vi "DRAM FIFO test with data.vi"() -> ()   [LabVIEW 2019]
uses:
  <instrlib>/FlexRIO/DRAM FIFO/v2/FPGA/DRAM FIFO/DRAM FIFO Status.ctl
  <instrlib>/FlexRIO/DRAM FIFO/v2/FPGA/DRAM FIFO/FIFO Depth.ctl
  <vilib>/Platform/TimedLoop/XDataNode/timing_clust.ctl
  <vilib>/Platform/TimedLoop/XDataNode/nitl_modes.ctl
  <vilib>/Platform/TimedLoop/XDataNode/wakeup.ctl
  <instrlib>/FlexRIO/DRAM FIFO/v2/FPGA/DRAM FIFO/dynamic arbitration select.ctl
  <instrlib>/FlexRIO/DRAM FIFO/v2/FPGA/DRAM FIFO/Private/DRAM FIFO U512/Create 512x1 DRAM FIFO.vi
  <vilib>/rvi/Emulation/niFpgaSctlEmulationGetInTimedLoop.vi
  <vilib>/rvi/Emulation/niFpgaEmulationReportErrorSimple.vi
  <vilib>/rvi/Emulation/niFpgaGetClockAttributes.vi
  <vilib>/rvi/Emulation/niFpgaCriticalErrorInLSC.vi
  <vilib>/rvi/Emulation/niFpgaProcessEmulError.vi
  <instrlib>/_niInstr/Basic Elements/v1/FPGA/Private/Count Up U32.vi
  <instrlib>/_niInstr/Basic Elements/v1/FPGA/Private/Count Up U16.vi
  <instrlib>/_niInstr/Data Formatting/v1/FPGA/Private/Convert/FXP(+-,12,1) array to Boolean Array.vi
  <instrlib>/_niInstr/Basic Elements/v1/FPGA/Private/Count Down U32.vi
  <instrlib>/FlexRIO/DRAM FIFO/v2/FPGA/DRAM FIFO/Pack Boolean Array.vi
  <vilib>/rvi/interface/RandomDataEmulation/nirviRandomDataMultiElementFPGAFIFO.vi
  <instcachedir>/0/nirviRandomDataMultiElementFPGAFIFO_1ED88BA00AC641F388A9B1FAA20E354D.lvgen/nirviRandomDataMultiElementFPGAFIFO_1ED88BA00AC641F388A9B1FAA20E354D_003.vi
  <vilib>/rvi/interface/RandomDataEmulation/niFpgaRandomDataHandleErrors.vi
  <vilib>/platform/TimedLoop/XDataNode/XDataNode.xnode
  <vilib>/rvi/FXPMathLib/FxpInterpret/XNode/nifxpmath_Interpret.xnode
  <vilib>/rvi/DataTransferAndStorage/Container/XNode/niFpgaContainer.xnode
  <vilib>/rvi/interface/RandomDataEmulation/nirviRandomDataFpgaMultiElementTemplate.vi
  <instrlib>/FlexRIO/DRAM FIFO/v2/FPGA/DRAM FIFO/DRAM FIFO v2 FPGA.lvclass
  <vilib>/Platform/TimedLoop/XDataNode/XDNodeRunTimeDep.lvlib
  <instrlib>/_niInstr/Data Formatting/v1/FPGA/niInstr Data Formatting v1 FPGA.lvlib
  <instrlib>/_niInstr/Basic Elements/v1/FPGA/niInstr Basic Elements v1 FPGA.lvlib
  SubVIs/Utility/FPGA Utility.lvlib
  <instrlib>/FlexRIO/DRAM FIFO/v2/FPGA/DRAM FIFO/Private/DRAM FIFO U512/DRAM FIFO U512 v2 FPGA.lvclass
panel:
  out "DRAM writes ctr":u32
  out "dram full latch":bool
  out "DRAM highwater 2":u32
  out "acq active":bool
  in  "start":bool
  in  "signal length":u32
  out "DRAM overflow":bool
  out "DRAM highwater":u32
  out "reset in progress?":bool
  in  "reset DRAM":bool
  out "status":T1
  in  "reset":bool
  in  "dram.flush":bool
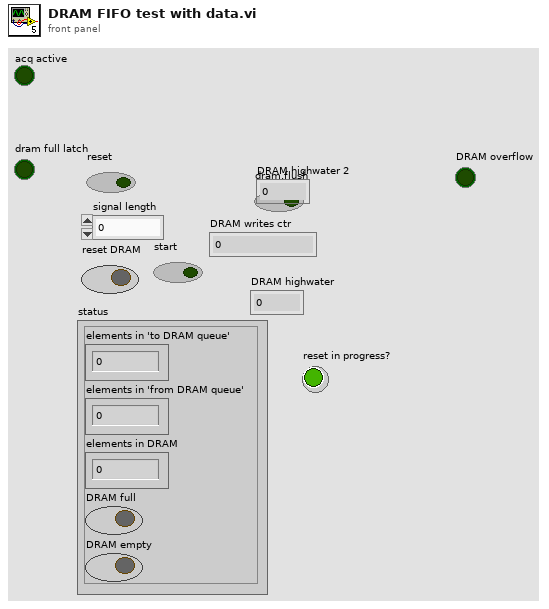
[diagram p1: front panel]
types:
  T1 = typedef "DRAM FIFO v2 FPGA.lvclass/DRAM FIFO Status.ctl" = cluster{"elements in 'to DRAM queue'":u32, "elements in 'from DRAM queue'":u32, "elements in DRAM":u32, "DRAM full":bool, "DRAM empty":bool}
  T2 = typedef "DRAM FIFO v2 FPGA.lvclass/FIFO Depth.ctl" = u8
  T3 = typedef "XDNodeRunTimeDep.lvlib/timing_clust.ctl" = cluster{"Expected End [f-1]":u64, "Actual End [f-1]":u64, "Finished Late? [f-1]":bool, "Expected End [i-1]":u64, "Actual End [i-1]":u64, "Finished Late? [i-1]":bool, "Expected Start [i]":u64, "Actual Start [i]":u64, "Expected Start [f]":u64, "Actual Start [f]":u64, "Source Name":string, "Structure Name":string, "Period":i64, "Deadline":i64, "Offset":i64, "Start":i64, "Priority":i32, "Timeout":i32, "Mode":T4, "Wakeup Reason":T5, "Error":errorcluster, "Source Type":string, "Secondary Source Type":string, "Global End Time":u64, "Global Start Time":u64, "Frame Duration":u64, "Iteration Duration":u64, "Assigned CPU":i32, "I/O Scan Engine Mode":u32}
  T4 = typedef "XDNodeRunTimeDep.lvlib/nitl_modes.ctl" = enum32{"No Change", "Process missed periods, maintain original phase", "Discard missed periods, maintain original phase", "Process missed periods, ignore original phase", "Discard missed periods, ignore original phase"}
  T5 = typedef "XDNodeRunTimeDep.lvlib/wakeup.ctl" = enum32{"Normal", "Aborted", "Asynchronous wakeup", "Timing source error", "Timed loop error", "Timeout"}
  T6 = typedef "DRAM FIFO v2 FPGA.lvclass/dynamic arbitration select.ctl" = enum16{"none", "dynamic (priority writes)", "dynamic (priority reads)"}
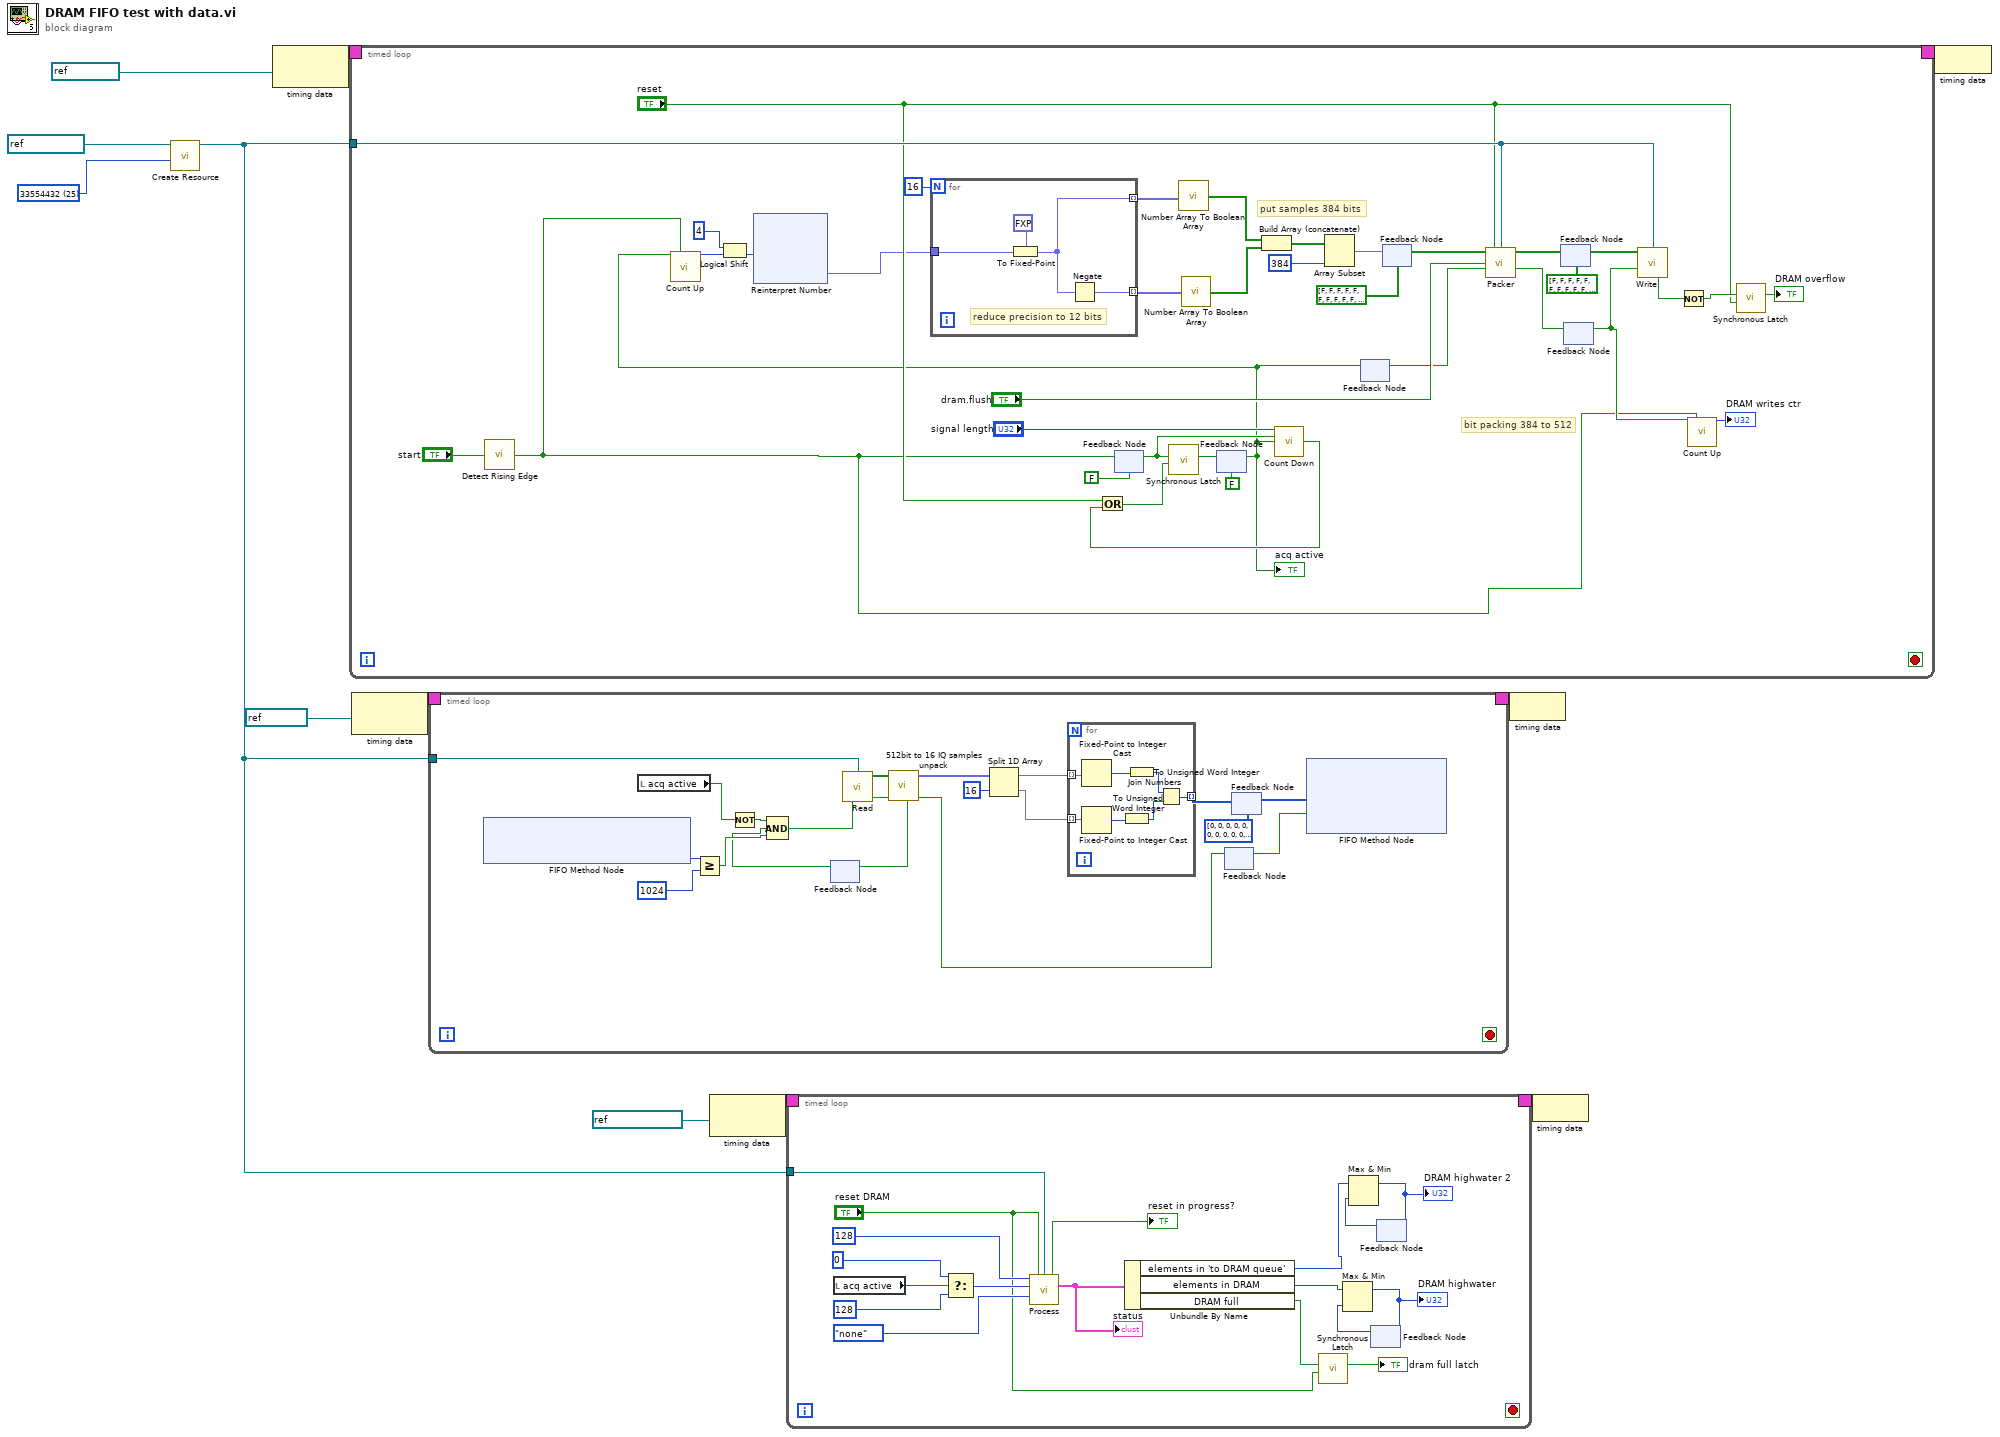
[diagram p0: block diagram]
diagram:
  w9 = T2 25 items=["4"=2, "8"=3, "16"=4, "32"=5, "64"=6, "128"=7, "256"=8, "512"=9, "1024"=10, "2048"=11, "4096"=12, "8192"=13, "16384"=14, "32768"=15, "65536"=16, "131072"=17, "262144"=18, "524288"=19, "1048576"=20, "2097152"=21, "4194304"=22, "8388608"=23, "16777216"=24, "33554432"=25, "67108864"=26, "134217728"=27, "268435456"=28, "536870912"=29, "1073741824"=30, "2147483648"=31, "4294967296"=32] ("actual # of DRAM elements")
  n1 = call-poly <instrlib>:"Create Resource.vi"("actual # of DRAM elements"=w9, "memory refnum"=refnum<k21> "RX memo") -> ("DRAM FIFO ref out"=w1:refnum<class "DRAM FIFO v2 FPGA.lvclass">)  [unwired: 9 in]
  n2 = node-c288(refnum<k21> "192MHz" ("Source Name")) -> (w7:T3)
  n3 = timed-loop {
    timing: w7 -> [_]
    timing-out: [_] -> w6
    tunnel: w1 -> [w32]
    stop <- _ stop-if-true
    # "bit packing 384 to 512"
    # "put samples 384 bits"
    n4 = call <instrlib>:"Detect Rising Edge.vi"("signal"="start") -> ("edge detected"=w14:bool)  [unwired: 14 in]
    n5 = feedback #1(FALSE ("edge detected")) -> (w36:bool)
    n6 = feedback-in #1(w14) -> ()
    n7 = feedback #2(FALSE ("out")) -> (w21:bool)
    "acq active" <- w21
    n8 = call-poly <instrlib>:"Count Up.vi"("increment"=w21, "reset"=w14) -> ("count out"=w19:u16)  [unwired: 13 in]
    n9 = Logical Shift(y=i16 4, x=w19) -> (x << y=w17:u16)
    n10 = xnode "Reinterpret Number"("x"=w17) -> ("y"=w18:fxp<+/-,16,1>)
    n11 = for {
      N: 16 -> [_]
      tunnel: [w50] -> w46 mode=indexing
      tunnel: [w52] -> w42 mode=indexing
      tunnel: w18 -> [w51]
      # "reduce precision to 12 bits"
      n12 = To Fixed-Point(fixed-point type=fxp<+/-,12,1> 0.0, number=w51) -> (fixed-point=w50:fxp<+/-,12,1>)
      n13 = Negate(x=w50) -> (-x=w52:fxp<+/-,12,1>)
    }
    n14 = call-poly <instrlib>:"Number Array To Boolean Array.vi"("data in"=w46) -> ("data out"=w45:bool[])  [unwired: 14 in]
    n15 = call-poly <instrlib>:"Number Array To Boolean Array.vi"("data in"=w42) -> ("data out"=w41:bool[])  [unwired: 14 in]
    n16 = Build Array (concatenate)(w45, w41) -> (w43:bool[])
    n17 = call-poly <instrlib>:"Count Down.vi"("count in"="signal length", "load"=w36, "decrement"=w21) -> ("terminal count"=w31:bool)  [unwired: 11 in, 1 out]
    n18 = Or(x="reset", y=w31) -> (x .or. y?=w30:bool)
    n19 = call <instrlib>:"Synchronous Latch.vi"("clear"=w30, "set"=w36) -> ("out"=w29:bool)  [unwired: 9 in]
    n20 = feedback-in #2(w29) -> ()
    n21 = Array Subset(array=w43, length=384) -> (w28:bool[])  [unwired: 1 in]
    n22 = feedback #3() -> (w25:bool)  [unwired: 1 in]
    n23 = feedback-in #3(w21) -> ()
    n24 = feedback #4(bool[] [FALSE, FALSE, FALSE, FALSE, FALSE, FALSE, FALSE, FALSE, FALSE, FALSE, FALSE, FALSE, FALSE, FALSE, FALSE, FALSE, FALSE, FALSE, FALSE, FALSE, FALSE, FALSE, FALSE, FALSE, FALSE, FALSE, FALSE, FALSE, FALSE, FALSE, FALSE, FALSE, FALSE, FALSE, FALSE, FALSE, FALSE, FALSE, FALSE, FALSE, FALSE, FALSE, FALSE, FALSE, FALSE, FALSE, FALSE, FALSE, FALSE, FALSE, FALSE, FALSE, FALSE, FALSE, FALSE, FALSE, FALSE, FALSE, FALSE, FALSE, FALSE, FALSE, FALSE, FALSE, FALSE, FALSE, FALSE, FALSE, FALSE, FALSE, FALSE, FALSE, FALSE, FALSE, FALSE, FALSE, FALSE, FALSE, FALSE, FALSE, FALSE, FALSE, FALSE, FALSE, FALSE, FALSE, FALSE, FALSE, FALSE, FALSE, FALSE, FALSE, FALSE, FALSE, FALSE, FALSE, FALSE, FALSE, FALSE, FALSE, FALSE, FALSE, FALSE, FALSE, FALSE, FALSE, FALSE, FALSE, FALSE, FALSE, FALSE, FALSE, FALSE, FALSE, FALSE, FALSE, FALSE, FALSE, FALSE, FALSE, FALSE, FALSE, FALSE, FALSE, FALSE, FALSE, FALSE, FALSE, FALSE, FALSE, FALSE, FALSE, FALSE, FALSE, FALSE, FALSE, FALSE, FALSE, FALSE, FALSE, FALSE, FALSE, FALSE, FALSE, FALSE, FALSE, FALSE, FALSE, FALSE, FALSE, FALSE, FALSE, FALSE, FALSE, FALSE, FALSE, FALSE, FALSE, FALSE, FALSE, FALSE, FALSE, FALSE, FALSE, FALSE, FALSE, FALSE, FALSE, FALSE, FALSE, FALSE, FALSE, FALSE, FALSE, FALSE, FALSE, FALSE, FALSE, FALSE, FALSE, FALSE, FALSE, FALSE, FALSE, FALSE, FALSE, FALSE, FALSE, FALSE, FALSE, FALSE, FALSE, FALSE, FALSE, FALSE, FALSE, FALSE, FALSE, FALSE, FALSE, FALSE, FALSE, FALSE, FALSE, FALSE, FALSE, FALSE, FALSE, FALSE, FALSE, FALSE, FALSE, FALSE, FALSE, FALSE, FALSE, FALSE, FALSE, FALSE, FALSE, FALSE, FALSE, FALSE, FALSE, FALSE, FALSE, FALSE, FALSE, FALSE, FALSE, FALSE, FALSE, FALSE, FALSE, FALSE, FALSE, FALSE, FALSE, FALSE, FALSE, FALSE, FALSE, FALSE, FALSE, FALSE, FALSE, FALSE, FALSE, FALSE, FALSE, FALSE, FALSE, FALSE, FALSE, FALSE, FALSE, FALSE, FALSE, FALSE, FALSE, FALSE, FALSE, FALSE, FALSE, FALSE, FALSE, FALSE, FALSE, FALSE, FALSE, FALSE, FALSE, FALSE, FALSE, FALSE, FALSE, FALSE, FALSE, FALSE, FALSE, FALSE, FALSE, FALSE, FALSE, FALSE, FALSE, FALSE, FALSE, FALSE, FALSE, FALSE, FALSE, FALSE, FALSE, FALSE, FALSE, FALSE, FALSE, FALSE, FALSE, FALSE, FALSE, FALSE, FALSE, FALSE, FALSE, FALSE, FALSE, FALSE, FALSE, FALSE, FALSE, FALSE, FALSE, FALSE, FALSE, FALSE, FALSE, FALSE, FALSE, FALSE, FALSE, FALSE, FALSE, FALSE, FALSE, FALSE, FALSE, FALSE, FALSE, FALSE, FALSE, FALSE, FALSE, FALSE, FALSE, FALSE, FALSE, FALSE, FALSE, FALSE, FALSE, FALSE, FALSE, FALSE, FALSE, FALSE, FALSE, FALSE, FALSE, FALSE, FALSE, FALSE, FALSE, FALSE, FALSE, FALSE, FALSE, FALSE, FALSE, FALSE, FALSE, FALSE, FALSE, FALSE, FALSE, FALSE, FALSE, FALSE, FALSE, FALSE, FALSE, FALSE, FALSE, FALSE, FALSE, FALSE, FALSE, FALSE, FALSE, FALSE, FALSE, FALSE, FALSE]) -> (w27:bool[])
    n25 = feedback-in #4(w28) -> ()
    n26 = call-poly <instrlib>:"Packer.vi"("data in"=w27, "reset"="reset", "DRAM FIFO in"=w32, "flush data"="dram.flush", "input valid"=w25) -> ("data out"=w47:bool[], "output valid"=w48:bool)  [unwired: 8 in, 1 out]
    n27 = feedback #5(bool[] [FALSE, FALSE, FALSE, FALSE, FALSE, FALSE, FALSE, FALSE, FALSE, FALSE, FALSE, FALSE, FALSE, FALSE, FALSE, FALSE, FALSE, FALSE, FALSE, FALSE, FALSE, FALSE, FALSE, FALSE, FALSE, FALSE, FALSE, FALSE, FALSE, FALSE, FALSE, FALSE, FALSE, FALSE, FALSE, FALSE, FALSE, FALSE, FALSE, FALSE, FALSE, FALSE, FALSE, FALSE, FALSE, FALSE, FALSE, FALSE, FALSE, FALSE, FALSE, FALSE, FALSE, FALSE, FALSE, FALSE, FALSE, FALSE, FALSE, FALSE, FALSE, FALSE, FALSE, FALSE, FALSE, FALSE, FALSE, FALSE, FALSE, FALSE, FALSE, FALSE, FALSE, FALSE, FALSE, FALSE, FALSE, FALSE, FALSE, FALSE, FALSE, FALSE, FALSE, FALSE, FALSE, FALSE, FALSE, FALSE, FALSE, FALSE, FALSE, FALSE, FALSE, FALSE, FALSE, FALSE, FALSE, FALSE, FALSE, FALSE, FALSE, FALSE, FALSE, FALSE, FALSE, FALSE, FALSE, FALSE, FALSE, FALSE, FALSE, FALSE, FALSE, FALSE, FALSE, FALSE, FALSE, FALSE, FALSE, FALSE, FALSE, FALSE, FALSE, FALSE, FALSE, FALSE, FALSE, FALSE, FALSE, FALSE, FALSE, FALSE, FALSE, FALSE, FALSE, FALSE, FALSE, FALSE, FALSE, FALSE, FALSE, FALSE, FALSE, FALSE, FALSE, FALSE, FALSE, FALSE, FALSE, FALSE, FALSE, FALSE, FALSE, FALSE, FALSE, FALSE, FALSE, FALSE, FALSE, FALSE, FALSE, FALSE, FALSE, FALSE, FALSE, FALSE, FALSE, FALSE, FALSE, FALSE, FALSE, FALSE, FALSE, FALSE, FALSE, FALSE, FALSE, FALSE, FALSE, FALSE, FALSE, FALSE, FALSE, FALSE, FALSE, FALSE, FALSE, FALSE, FALSE, FALSE, FALSE, FALSE, FALSE, FALSE, FALSE, FALSE, FALSE, FALSE, FALSE, FALSE, FALSE, FALSE, FALSE, FALSE, FALSE, FALSE, FALSE, FALSE, FALSE, FALSE, FALSE, FALSE, FALSE, FALSE, FALSE, FALSE, FALSE, FALSE, FALSE, FALSE, FALSE, FALSE, FALSE, FALSE, FALSE, FALSE, FALSE, FALSE, FALSE, FALSE, FALSE, FALSE, FALSE, FALSE, FALSE, FALSE, FALSE, FALSE, FALSE, FALSE, FALSE, FALSE, FALSE, FALSE, FALSE, FALSE, FALSE, FALSE, FALSE, FALSE, FALSE, FALSE, FALSE, FALSE, FALSE, FALSE, FALSE, FALSE, FALSE, FALSE, FALSE, FALSE, FALSE, FALSE, FALSE, FALSE, FALSE, FALSE, FALSE, FALSE, FALSE, FALSE, FALSE, FALSE, FALSE, FALSE, FALSE, FALSE, FALSE, FALSE, FALSE, FALSE, FALSE, FALSE, FALSE, FALSE, FALSE, FALSE, FALSE, FALSE, FALSE, FALSE, FALSE, FALSE, FALSE, FALSE, FALSE, FALSE, FALSE, FALSE, FALSE, FALSE, FALSE, FALSE, FALSE, FALSE, FALSE, FALSE, FALSE, FALSE, FALSE, FALSE, FALSE, FALSE, FALSE, FALSE, FALSE, FALSE, FALSE, FALSE, FALSE, FALSE, FALSE, FALSE, FALSE, FALSE, FALSE, FALSE, FALSE, FALSE, FALSE, FALSE, FALSE, FALSE, FALSE, FALSE, FALSE, FALSE, FALSE, FALSE, FALSE, FALSE, FALSE, FALSE, FALSE, FALSE, FALSE, FALSE, FALSE, FALSE, FALSE, FALSE, FALSE, FALSE, FALSE, FALSE, FALSE, FALSE, FALSE, FALSE, FALSE, FALSE, FALSE, FALSE, FALSE, FALSE, FALSE, FALSE, FALSE, FALSE, FALSE, FALSE, FALSE, FALSE, FALSE, FALSE, FALSE, FALSE, FALSE, FALSE, FALSE, FALSE, FALSE, FALSE, FALSE, FALSE, FALSE, FALSE, FALSE, FALSE, FALSE, FALSE, FALSE, FALSE, FALSE, FALSE, FALSE, FALSE, FALSE, FALSE, FALSE, FALSE, FALSE, FALSE, FALSE, FALSE, FALSE, FALSE, FALSE, FALSE, FALSE, FALSE, FALSE, FALSE, FALSE, FALSE, FALSE, FALSE, FALSE, FALSE, FALSE, FALSE, FALSE, FALSE, FALSE, FALSE, FALSE, FALSE, FALSE, FALSE, FALSE, FALSE, FALSE, FALSE, FALSE, FALSE, FALSE, FALSE, FALSE, FALSE, FALSE, FALSE, FALSE, FALSE, FALSE, FALSE, FALSE, FALSE, FALSE, FALSE, FALSE, FALSE, FALSE, FALSE, FALSE, FALSE, FALSE, FALSE, FALSE, FALSE, FALSE, FALSE, FALSE, FALSE, FALSE, FALSE, FALSE, FALSE, FALSE, FALSE, FALSE, FALSE, FALSE, FALSE, FALSE, FALSE, FALSE, FALSE, FALSE, FALSE, FALSE, FALSE, FALSE, FALSE, FALSE, FALSE, FALSE, FALSE, FALSE, FALSE, FALSE, FALSE, FALSE, FALSE, FALSE, FALSE, FALSE, FALSE, FALSE, FALSE, FALSE, FALSE, FALSE, FALSE, FALSE, FALSE, FALSE, FALSE, FALSE, FALSE, FALSE, FALSE]) -> (w24:bool[])
    n28 = feedback-in #5(w47) -> ()
    n29 = feedback #6() -> (w15:bool)  [unwired: 1 in]
    n30 = feedback-in #6(w48) -> ()
    n31 = call <instrlib>:"Write.vi"("element"=w24, "DRAM FIFO ref in"=w32, "input valid"=w15) -> ("ready for input"=w40:bool)  [unwired: 12 in]
    n32 = Not(x=w40) -> (.not. x?=w39:bool)
    n33 = call-poly <instrlib>:"Count Up.vi"("increment"=w15, "reset"=w14) -> ("count out"=→"DRAM writes ctr":u32)  [unwired: 13 in]
    n34 = call <instrlib>:"Synchronous Latch.vi"("clear"="reset", "set"=w39) -> ("out"=→"DRAM overflow":bool)  [unwired: 9 in]
  }
  n35 = node-c288(refnum<k21> "50MHz" ("Source Name")) -> (w4:T3)
  n36 = timed-loop {
    timing: w4 -> [_]
    timing-out: [_] -> w3
    tunnel: w1 -> [w59]
    stop <- _ stop-if-true
    n37 = xnode ("FIFO Method Node")() -> ("Number of Elements to Write"=w70:u32)  [unwired: 1 in, 1 out]
    n38 = local read "acq active"() -> (w58:bool)
    n39 = Greater Or Equal?(x=w70, y=u32 1024) -> (x >= y?=w72:bool)
    n40 = Not(x=w58) -> (.not. x?=w61:bool)
    n41 = feedback #7() -> (w62:bool)  [unwired: 1 in]
    n42 = Compound Arithmetic op=AND(w61, w62, w72) -> (w63:bool)
    n43 = call <instrlib>:"Read.vi"("DRAM FIFO ref in"=w59, "ready for output"=w63) -> ("element"=w64:bool[], "output valid"=w65:bool)  [unwired: 12 in]
    n44 = call "512bit to 16 IQ samples unpack.vi"("input valid"=w65, "data in"=w64) -> ("output valid"=w74:bool, "data out"=w67:fxp<+/-,12,1>[], "ready for input"=w66:bool)  [unwired: 7 in]
    n45 = feedback-in #7(w66) -> ()
    n46 = Split 1D Array(array=w67, index=16) -> (first subarray=w68:fxp<+/-,12,1>[], second subarray=w69:fxp<+/-,12,1>[])
    n47 = for {
      tunnel: w68 -> [w80] mode=indexing
      tunnel: w69 -> [w78] mode=indexing
      tunnel: [w82] -> w73 mode=indexing
      n48 = Fixed-Point to Integer Cast(1:w80) -> (0:w81:i16)
      n49 = Fixed-Point to Integer Cast(1:w78) -> (0:w79:i16)
      n50 = To Unsigned Word Integer(number=w79) -> (unsigned 16bit integer=w77:u16)
      n51 = To Unsigned Word Integer(number=w81) -> (unsigned 16bit integer=w76:u16)
      n52 = Join Numbers(hi=w76, lo=w77) -> ((hi.lo)=w82:u32)
    }
    n53 = feedback #8() -> (w75:bool)  [unwired: 1 in]
    n54 = feedback-in #8(w74) -> ()
    n55 = feedback #9(u32[] [0, 0, 0, 0, 0, 0, 0, 0, 0, 0, 0, 0, 0, 0, 0, 0] ("Element")) -> (w56:u32[])
    n56 = feedback-in #9(w73) -> ()
    n57 = xnode ("FIFO Method Node")("Element"=w56, "Input Valid"=w75) -> ()  [unwired: 1 in, 2 out]
  }
  n58 = node-c288(refnum<k21> "DRAM Clock" ("Source Name")) -> (w12:T3)
  n59 = timed-loop {
    timing: w12 -> [_]
    timing-out: [_] -> w11
    tunnel: w1 -> [w100]
    stop <- _ stop-if-true
    n60 = local read "acq active"() -> (w93:bool)
    n61 = Select(t=u16 0 ("read grant time (clock ticks)"), s=w93, f=u16 128 ("read grant time (clock ticks)")) -> (s? t:f=w91:u16)
    n62 = call <instrlib>:"Process.vi"("write grant time (clock ticks)"=u16 128, "reset DRAM"="reset DRAM", "DRAM FIFO ref in"=w100, "read grant time (clock ticks)"=w91, "dynamic arbitration"=dynamic_arbitration_select."none") -> ("reset in progress?"=→"reset in progress?":bool, "status"=w98:T1)  [unwired: 9 in]
    "status" <- w98
    n63 = Unbundle By Name(w98) -> ("elements in 'to DRAM queue'"=w89:u32, "elements in DRAM"=w97:u32, "DRAM full"=w87:bool)
    n64 = call <instrlib>:"Synchronous Latch.vi"("clear"="reset DRAM", "set"=w87) -> ("out"=→"dram full latch":bool)  [unwired: 9 in]
    n65 = feedback #10() -> (w95:u32)  [unwired: 1 in]
    n66 = Max & Min(x=w97, y=w95) -> (max(x,y)=w96:u32)  [unwired: 1 out]
    "DRAM highwater" <- w96
    n67 = feedback-in #10(w96) -> ()
    n68 = feedback #11() -> (w88:u32)  [unwired: 1 in]
    n69 = Max & Min(x=w89, y=w88) -> (max(x,y)=w90:u32)  [unwired: 1 out]
    "DRAM highwater 2" <- w90
    n70 = feedback-in #11(w90) -> ()
  }
  n71 = node-c288(w3) -> ()
  n72 = node-c288(w11) -> ()
  n73 = node-c288(w6) -> ()
